vi "nanoWatts_to_dBm.vi"(10 "P(nW)":dbl) -> (2 "dBm":dbl)   [LabVIEW 2018]
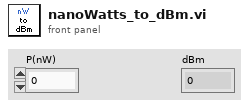
[diagram p1: front panel]
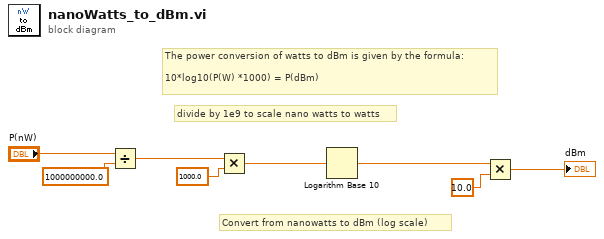
[diagram p0: block diagram]
diagram:
  # "divide by 1e9 to scale nano watts to watts"
  # "Convert from nanowatts to dBm (log scale)"
  # "The power conversion of watts to dBm is given by the formula:\n\n10*log10(P(W) *1000) = P(dBm)"
  n1 = Divide(x="P(nW)", y=1000000000.0) -> (x/y=w4:dbl)
  n2 = Multiply(x=w4, y=1000.0) -> (x*y=w7:dbl)
  n3 = Logarithm Base 10(1:w7) -> (0:w6:dbl)
  n4 = Multiply(x=w6, y=10.0) -> (x*y=→"dBm":dbl)
